vi "CTL_Spec LUT.vi"(6 "Max Index":i32=12, 8 "Level IN inches":dbl=5.0, 9 "Index":i32=3, 10 "ChA/!ChB":bool, 11 "Full Cfg":T3={"Bench Config"={"Name"="OLR001", {"Step Levels"=0.05, "Tolerance"=0.01, "Sample Rate"=0.05, "Resistor"=100.0, "M Level Cal"=1.0, "[B Level Cal"=0.0, "Max Fill Rate"=0.025, "Empty Inches"=8.6, "Full Inches"=2.0}}, "Test Value Table "=[[98.0, 102.0, 7.91, 8.01, 7.55, 7.65, 98.0, 102.0, 7.685, 7.785, 7.325, 7.425], [197.0, 203.0, 7.46, 7.56, 7.1, 7.2, 197.0, 203.0, 7.235, 7.335, 6.875, 6.975], [296.0, 304.0, 7.01, 7.11, 6.65, 6.75, 296.0, 304.0, 6.785, 6.885, 6.425, 6.525], [395.0, 405.0, 6.56, 6.66, 6.2, 6.3, 395.0, 405.0, 6.335, 6.435, 5.975, 6.075], [494.0, 506.0, 6.11, 6.21, 5.75, 5.85, 494.0, 506.0, 5.885, 5.985, 5.525, 5.625], [593.0, 607.0, 5.66, 5.76, 5.3, 5.4, 593.0, 607.0, 5.435, 5.535, 5.075, 5.175], [692.0, 708.0, 5.21, 5.31, 4.85, 4.95, 692.0, 708.0, 4.985, 5.085, 4.625, 4.725], [791.0, 809.0, 4.76, 4.86, 4.4, 4.5, 791.0, 809.0, 4.535, 4.635, 4.175, 4.275], [890.0, 910.0, 4.31, 4.41, 3.95, 4.05, 890.0, 910.0, 4.085, 4.185, 3.725, 3.825], [989.0, 1011.0, 3.86, 3.96, 3.5, 3.6, 989.0, 1011.0, 3.635, 3.735, 3.275, 3.375], [1088.0, 1112.0, 3.41, 3.51, 3.05, 3.15, 1088.0, 1112.0, 3.185, 3.285, 2.825, 2.925], [0.0, 0.0, 0.0, 0.0, 0.0, 0.0, 0.0, 0.0, 0.0, 0.0, 0.0, 0.0]], "Table Col Titles"=[["Aohm Lo", "Aohm Hi", "A Fill Lo", "A Fill Hi", "A Drain Lo", "A Drain Hi", "Bohm Lo", "Bohm Hi", "B Fill Lo", "B Fill Hi", "B Drain Lo", "B Drain Hi"]], "Pump CtlRef In"={"Fill "=refnum, "Drain"=refnum, "Level PV"=refnum, "Flow Rate%"=refnum, "Run Test"=refnum, "Sim"=refnum, "Jog"=refnum, "Level SP"=refnum}, "Bench Status"={"Pump Status"=refnum, "Instrumnet\n Status"=refnum}}) -> (2 "Spec RNG":T1={"Specs"=[6.885, 6.785, 6.435, 304.0, 296.0], "Index(n)"=2, "LUT Status"={"ChA/!ChB"=FALSE, "Drain/!Fill"=FALSE, "In Range?"=TRUE, "Switch Range?"=FALSE, "Measure R?"=FALSE, "Vaild R?"=FALSE}, "Index(n-1)"=1}, 3 "In Range?":bool=TRUE)   [LabVIEW 2024]
uses:
  Control Definitions/Def FullCfg.ctl
  Control Definitions/Def BenchCfg.ctl
  Control Definitions/Def PumpCtlRefs.ctl
  Control Definitions/Def Bench Status.ctl
  Control Definitions/Ded LUT_Status.ctl
  Control Definitions/Ded Spec RNG.ctl
panel:
  in  "Test \nDrain!Fill":bool
  in  "Cluster":T2
  out "error out":errorcluster
  in  "error in (no error)":errorcluster
  in  "Cluster 3":T1
  # "In Range = TRUE when"
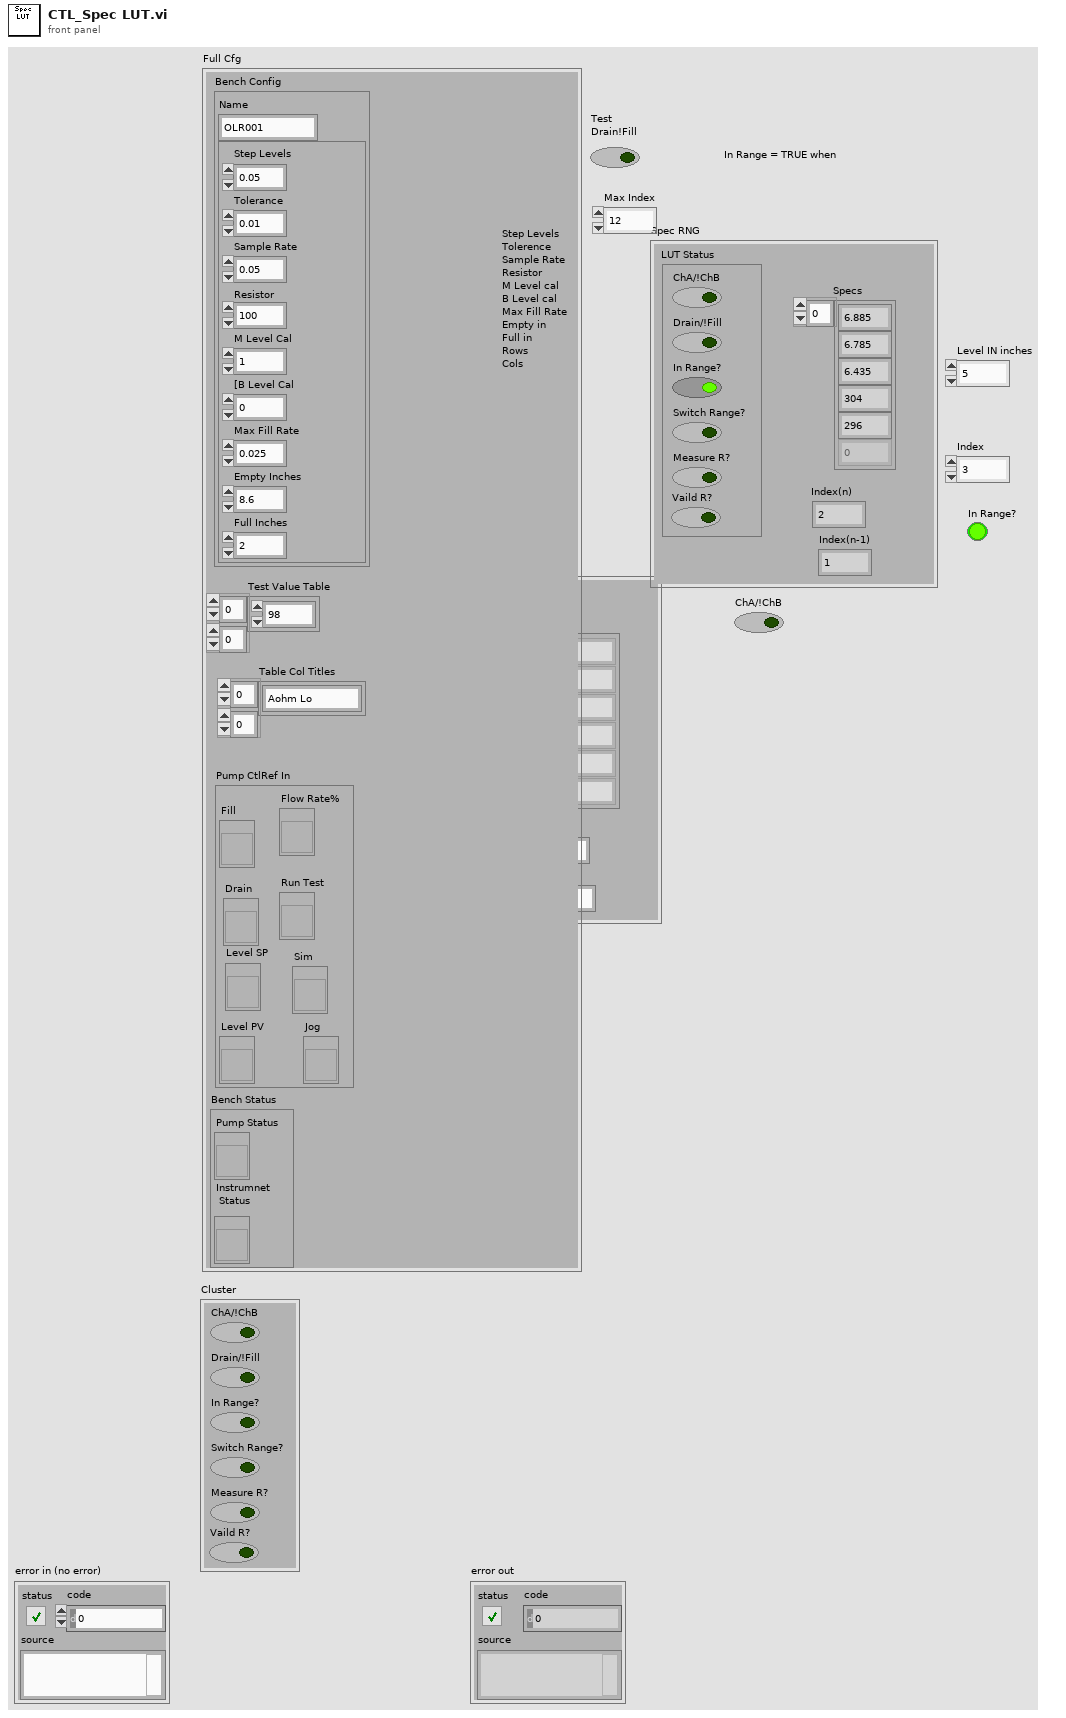
[diagram p1: front panel]
types:
  T1 = typedef "Ded Spec RNG.ctl" = cluster{"Specs":dbl[], "Index(n)":i32, "LUT Status":T2, "Index(n-1)":i32}
  T2 = typedef "Ded LUT_Status.ctl" = cluster{"ChA/!ChB":bool, "Drain/!Fill":bool, "In Range?":bool, "Switch Range?":bool, "Measure R?":bool, "Vaild R?":bool}
  T3 = typedef "Def FullCfg.ctl" = cluster{"Bench Config":T4, "Test Value Table ":dbl[][], "Table Col Titles":string[][], "Pump CtlRef In":T5, "Bench Status":T6}
  T4 = typedef "Def BenchCfg.ctl" = cluster{"Name":string, cluster{"Step Levels":dbl, "Tolerance":dbl, "Sample Rate":dbl, "Resistor":dbl, "M Level Cal":dbl, "[B Level Cal":dbl, "Max Fill Rate":dbl, "Empty Inches":dbl, "Full Inches":dbl}}
  T5 = typedef "Def PumpCtlRefs.ctl" = cluster{"Fill ":refnum<vi>, "Drain":refnum<vi>, "Level PV":refnum<vi>, "Flow Rate%":refnum<vi>, "Run Test":refnum<vi>, "Sim":refnum<vi>, "Jog":refnum<vi>, "Level SP":refnum<vi>}
  T6 = typedef "Def Bench Status.ctl" = cluster{"Pump Status":refnum<vi>, "Instrumnet\n Status":refnum<vi>}
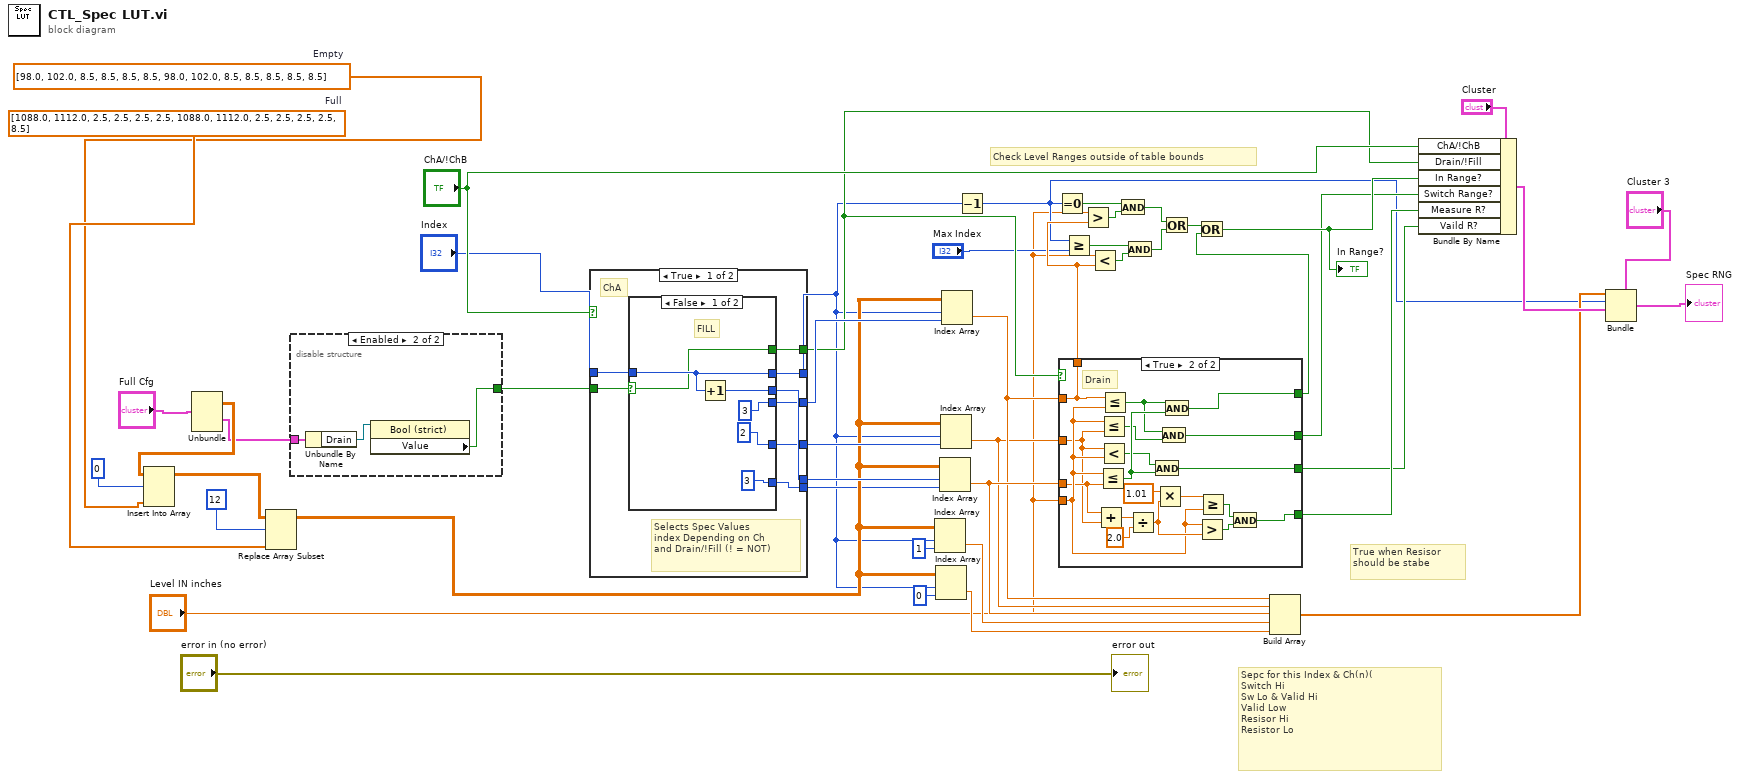
[diagram p0: block diagram]
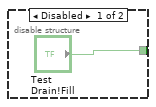
[diagram p2: hidden frame]
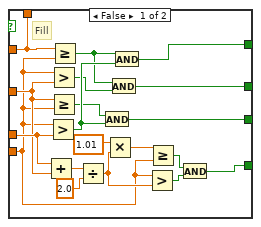
[diagram p3: hidden frame]
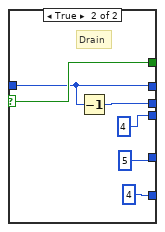
[diagram p4: hidden frame]
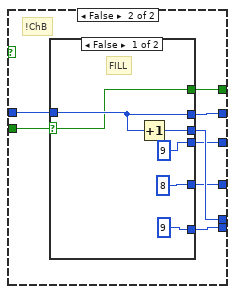
[diagram p5: hidden frame]
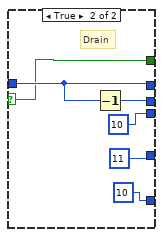
[diagram p6: hidden frame]
diagram:
  w16 = dbl[] [1088.0, 1112.0, 2.5, 2.5, 2.5, 2.5, 1088.0, 1112.0, 2.5, 2.5, 2.5, 2.5, 8.5]  # Full
  w9 = dbl[] [98.0, 102.0, 8.5, 8.5, 8.5, 8.5, 98.0, 102.0, 8.5, 8.5, 8.5, 8.5, 8.5]  # Empty
  # "True when Resisor \nshould be stabe"
  # "Sepc for this Index & Ch(n)(\nSwitch Hi\nSw Lo & Valid Hi  \nValid Low\nResisor Hi\nResistor Lo"
  # "Check Level Ranges outside of table bounds"
  n1 = Unbundle("Full Cfg") -> ("Test Value Table"=w8:dbl[][], "Pump CtlRef In"=w3:T5)  [unwired: 3 out]
  n2 = Insert Into Array(array=w8, index (row)=0 ("disabled index (col)"), new element=w9) -> (w7:dbl[][])  [unwired: 1 in]
  n3 = Replace Array Subset(array=w7, new element=w16, index (row)=12 ("disabled index (col)")) -> (w15:dbl[][])  [unwired: 1 in]
  n4 = disable-structure shown="Enabled" {
    disable-tunnel: w3 -> [_ w51]
    disable-tunnel: ["Test \nDrain!Fill" w49] -> w2
    frame Disabled {
    }
    frame Enabled {
      n5 = Unbundle By Name(w51) -> ("Drain"=w50:refnum<vi>)
      n6 = property class="Bool (strict)"(reference=w50) -> ("Value"=w49:bool)  [unwired: 1 in, 2 out]
    }
  }
  n7 = case shown="True" "ChA/!ChB" {
    tunnel: w2 -> [w59 w73]
    tunnel: "Index" -> [w58 w79]
    tunnel: [w57 w78] -> w5
    tunnel: [w56 w77] -> w44
    tunnel: [w55 w76] -> w43
    tunnel: [w54 w75] -> w42
    tunnel: [w53 w74] -> w11
    tunnel: [w52 w72] -> w25
    frame True {
      # "Selects Spec Values\nindex Depending on Ch\nand Drain/!Fill (! = NOT)"
      # "ChA"
      n8 = case shown="False" w59 {
        selector: w59 -> [w60 w68]
        tunnel: [3 ("disabled index (col)") 4 ("disabled index (col)")] -> w53
        tunnel: [3 ("disabled index (col)") 4 ("disabled index (col)")] -> w55
        tunnel: w58 -> [w61 w66]
        tunnel: [w61 w66] -> w57
        tunnel: [w63 w67] -> w56
        tunnel: [2 ("disabled index (col)") 5 ("disabled index (col)")] -> w54
        tunnel: [w60 w68] -> w52
        frame False {
          # "FILL"
          n9 = Increment(x=w61) -> (x+1=w63:i32)
        }
        frame True {
          # "Drain"
          n10 = Decrement(x=w66) -> (x-1=w67:i32)
        }
      }
    }
    frame False {
      # "!ChB"
      n11 = case shown="False" w73 {
        selector: w73 -> [w80 w86]
        tunnel: [9 ("disabled index (col)") 10 ("disabled index (col)")] -> w74
        tunnel: [9 ("disabled index (col)") 10 ("disabled index (col)")] -> w76
        tunnel: w79 -> [w81 w87]
        tunnel: [w81 w87] -> w78
        tunnel: [w83 w89] -> w77
        tunnel: [8 ("disabled index (col)") 11 ("disabled index (col)")] -> w75
        tunnel: [w80 w86] -> w72
        frame False {
          # "FILL"
          n12 = Increment(x=w81) -> (x+1=w83:i32)
        }
        frame True {
          # "Drain"
          n13 = Decrement(x=w87) -> (x-1=w89:i32)
        }
      }
    }
  }
  n14 = Index Array(array=w15, index (row)=w5, index (col)=1 ("disabled index (col)")) -> (element=w41:dbl)
  n15 = Index Array(array=w15, index (row)=w5, index (col)=0 ("disabled index (col)")) -> (element=w40:dbl)
  n16 = Index Array(array=w15, index (row)=w44, index (col)=w11) -> (element=w39:dbl)
  n17 = Index Array(array=w15, index (row)=w5, index (col)=w42) -> (element=w29:dbl)
  n18 = Index Array(array=w15, index (row)=w5, index (col)=w43) -> (element=w30:dbl)
  n19 = Decrement(x=w5) -> (x-1=w4:i32)
  n20 = Equal To 0?(x=w4) -> (x = 0?=w35:bool)
  n21 = case shown="True" w25 {
    tunnel: "Level IN inches" -> [w94 w115]
    tunnel: w30 -> [w92 w113]
    tunnel: w39 -> [w103 w112]
    tunnel: [w110 w129] -> w31
    tunnel: w29 -> [w102 w111]
    tunnel: [w107 w126] -> w19
    tunnel: [w104 w123] -> w23
    tunnel: [w93 w114] -> w22
    tunnel: [w92 w113] -> w13
    frame False {
      # "Fill"
      n22 = Add(x=w103, y=w102) -> (x+y=w101:dbl)
      n23 = Greater?(x=w94, y=w103) -> (0:w109:bool)
      n24 = Greater?(x=w94, y=w102) -> (0:w105:bool)
      n25 = Greater Or Equal?(x=w102, y=w94) -> (x >= y?=w108:bool)
      n26 = Greater Or Equal?(x=w92, y=w94) -> (x >= y?=w106:bool)
      n27 = Divide(x=w101, y=2.0) -> (x/y=w95:dbl)
      n28 = And(x=w108, y=w109) -> (x .and. y?=w107:bool)
      n29 = Multiply(x=1.01, y=w95) -> (x*y=w96:dbl)
      n30 = And(x=w106, y=w105) -> (x .and. y?=w104:bool)
      n31 = And(x=w106, y=w109) -> (x .and. y?=w110:bool)
      n32 = Greater?(x=w94, y=w95) -> (0:w99:bool)
      n33 = Greater Or Equal?(x=w96, y=w94) -> (x >= y?=w98:bool)
      n34 = And(x=w98, y=w99) -> (x .and. y?=w93:bool)
    }
    frame True {
      # "Drain"
      n35 = Add(x=w112, y=w111) -> (x+y=w122:dbl)
      n36 = Less Or Equal?(x=w115, y=w112) -> (x <= y?=w128:bool)
      n37 = Less Or Equal?(x=w115, y=w111) -> (x <= y?=w124:bool)
      n38 = Less?(x=w111, y=w115) -> (x < y?=w127:bool)
      n39 = Less Or Equal?(x=w113, y=w115) -> (x <= y?=w125:bool)
      n40 = Divide(x=w122, y=2.0) -> (x/y=w116:dbl)
      n41 = And(x=w127, y=w128) -> (x .and. y?=w126:bool)
      n42 = Multiply(x=1.01, y=w116) -> (x*y=w117:dbl)
      n43 = And(x=w125, y=w124) -> (x .and. y?=w123:bool)
      n44 = And(x=w125, y=w128) -> (x .and. y?=w129:bool)
      n45 = Greater?(x=w115, y=w116) -> (0:w120:bool)
      n46 = Greater Or Equal?(x=w117, y=w115) -> (x >= y?=w119:bool)
      n47 = And(x=w119, y=w120) -> (x .and. y?=w114:bool)
    }
  }
  n48 = Greater Or Equal?(x=w4, y="Max Index") -> (x >= y?=w37:bool)
  n49 = Greater?(x="Level IN inches", y=w13) -> (0:w36:bool)
  n50 = Less?(x="Level IN inches", y=w13) -> (x < y?=w38:bool)
  n51 = And(x=w35, y=w36) -> (x .and. y?=w33:bool)
  n52 = And(x=w37, y=w38) -> (x .and. y?=w34:bool)
  n53 = Or(x=w33, y=w34) -> (x .or. y?=w32:bool)
  n54 = Or(x=w32, y=w31) -> (x .or. y?=w24:bool)
  "In Range?" <- w24
  n55 = Build Array(w30, w29, w39, w41, w40) -> (w17:dbl[])
  n56 = Bundle By Name(cluster="Cluster", "ChA/!ChB"="ChA/!ChB", "Drain/!Fill"=w25, "In Range?"=w24, "Switch Range?"=w23, "Measure R?"=w22, "Vaild R?"=w19) -> (w18:T2)
  n57 = Bundle(cluster="Cluster 3", "Specs"=w17, "Index(n)"=w4, "LUT Status"=w18) -> (→"Spec RNG":T1)  [unwired: 1 in]
  "error out" <- "error in (no error)"
